vi "Stack_holderwise_total_bd_count_&_duration_ST1.vi"(0 "Refnum in":T1, 1 "BREAKDOWN_STK_HOLD_ID":i32=1, 2 "condition":string="Where BREAKDOWN_DATE between '%s'and '%s' and BREAKDOWN_STK_HOLD_ID ='%d'  ", 5 "Form Date":timestamp, 7 "Array":string[](array[string]), 9 "To Date":timestamp, 11 "error in (no error)":errorcluster, 12 "STATION_ID_CID_TRIGGER":i32, 13 "table":string[](array[string])=["STATION_1_LOG_HISTORY", "STATION_2_LOG_HISTORY", "STATION_3_LOG_HISTORY", "STATION_4_LOG_HISTORY", "STATION_5_LOG_HISTORY", "STATION_6_LOG_HISTORY"]) -> (4 "Refnum out":T1, 6 "Count out":string[](array[string]), 10 "appended array":dbl[](array[numeric]), 15 "error out":errorcluster)   [LabVIEW 2017]
uses:
  <vilib>/addons/database/Connection.llb/Conn ObjectReference.ctl
  <vilib>/addons/database/NI_Database_API.lvlib
panel:
  out "Table":string[][](array[string])
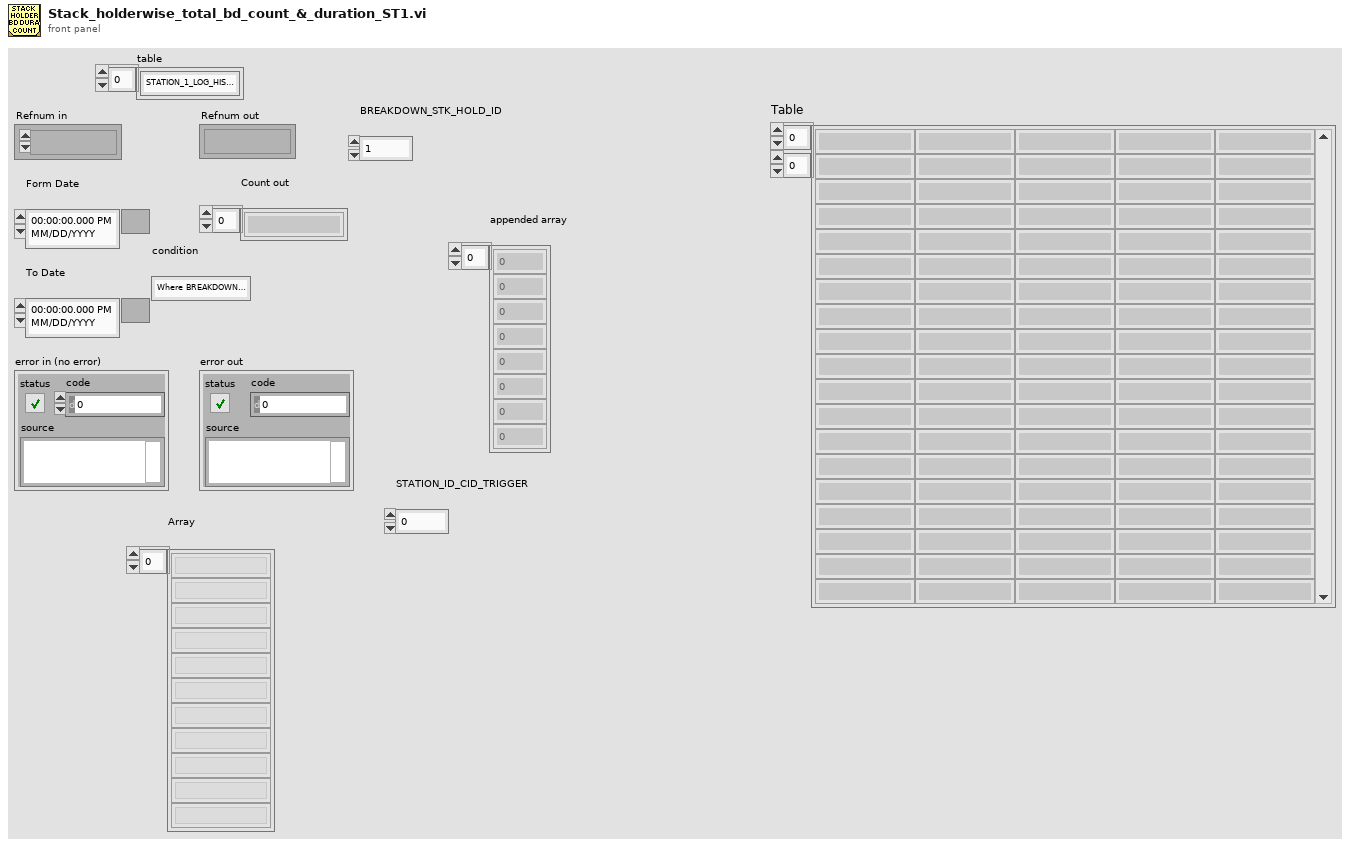
[diagram p1: front panel]
types:
  T1 = typedef "NI_Database_API.lvlib/Conn ObjectReference.ctl" = refnum<k1>
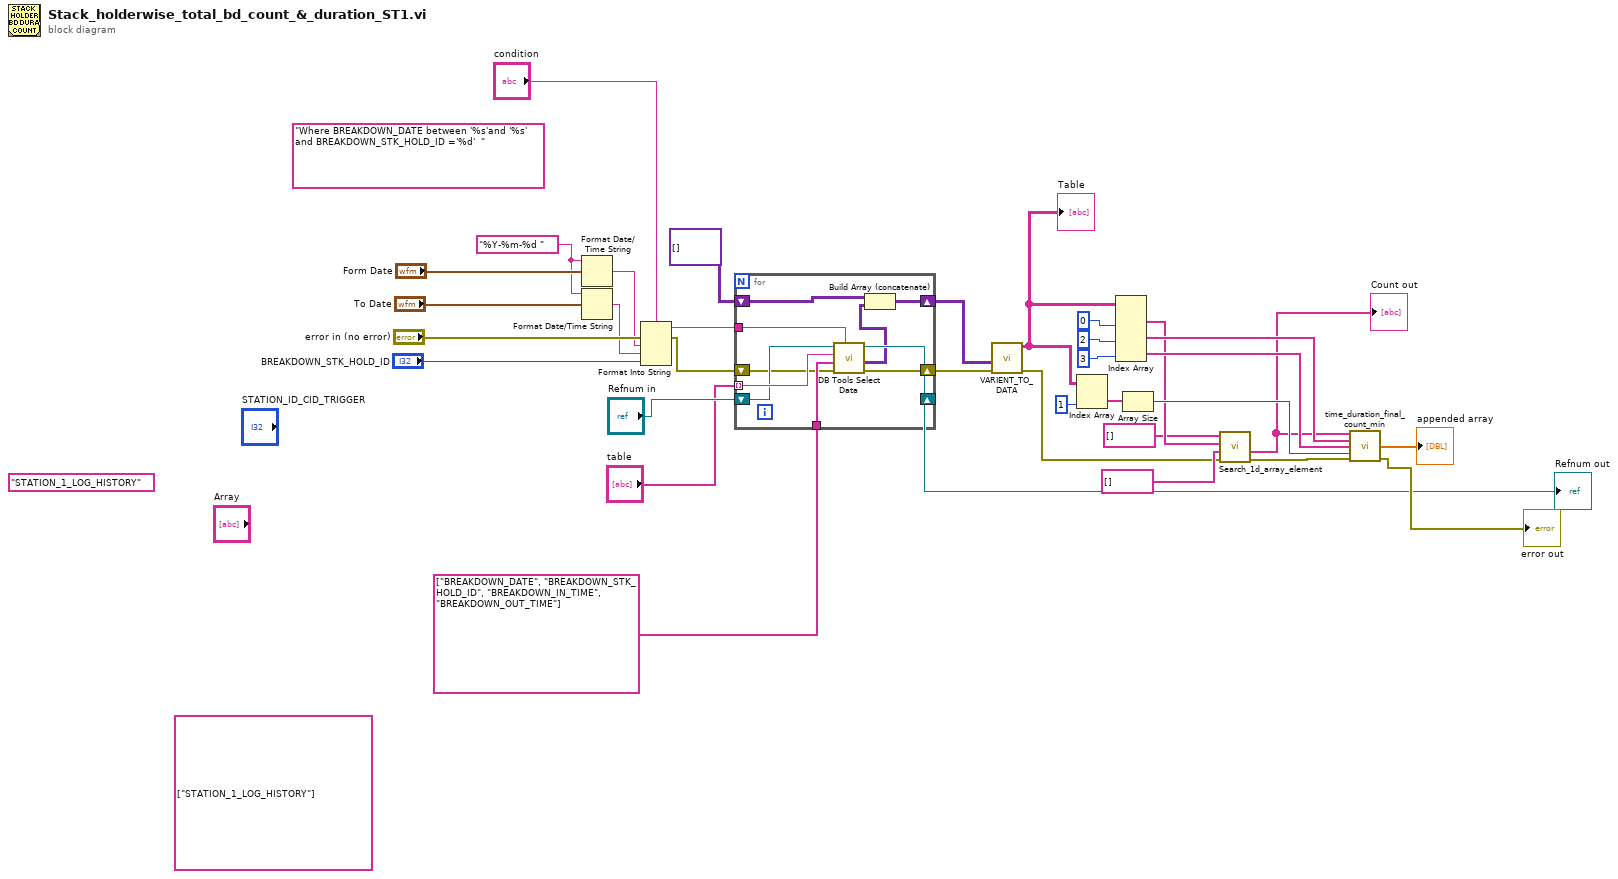
[diagram p0: block diagram]
diagram:
  (unwired) string[] ["STATION_1_LOG_HISTORY"]
  (unwired) "Where BREAKDOWN_DATE between '%s'and '%s' and BREAKDOWN_STK_HOLD_ID ='%d'  "
  (unwired) "STATION_1_LOG_HISTORY" ("table")
  w10 = "%Y-%m-%d " ("time format string (%c)")
  n1 = Format Date/Time String(time format string (%c)=w10, seconds (now)="Form Date") -> (date/time string=w13:string)  [unwired: 1 in]
  n2 = Format Date/Time String(time format string (%c)=w10, seconds (now)="To Date") -> (date/time string=w14:string)  [unwired: 1 in]
  n3 = Format Into String(format string="condition", error in="error in (no error)", w13, w14, "BREAKDOWN_STK_HOLD_ID") -> (resulting string=w6:string, error out=w7:errorcluster)  [unwired: 1 in]
  n4 = for {
    tunnel: "table" -> [w44] mode=indexing
    tunnel: string[] ["BREAKDOWN_DATE", "BREAKDOWN_STK_HOLD_ID", "BREAKDOWN_IN_TIME", "BREAKDOWN_OUT_TIME"] -> [w43]
    tunnel: w6 -> [w38]
    shift-right: [w42] -> w17
    shift-left: "Refnum in" -> [w41]
    shift-right: [w40] -> w8
    shift-left: w7 -> [w39]
    shift-right: [w35] -> w9
    shift-left: variant[][] [] ("data") -> [w37]
    n5 = call <vilib>:"DB Tools Select Data.vi"("condition"=w38, "error in (no error)"=w39, "columns"=w43, "table"=w44, "connection reference"=w41) -> ("error out"=w40:errorcluster, "data"=w36:variant[][], "connection reference out"=w42:T1)  [unwired: 1 in]
    n6 = Build Array (concatenate)(w37, w36) -> (w35:variant[][])
  }
  "Refnum out" <- w17
  n7 = call "VARIENT_TO_DATA.vi"("data"=w9, "error in (no error)"=w8) -> ("Table"=w31:string[][], "error out"=w32:errorcluster)  [unwired: 7 in]
  "Table" <- w31
  n8 = Index Array(array=w31, index (col)=1 ("disabled index (col)")) -> (element=w24:string[])  [unwired: 1 in]
  n9 = Index Array(array=w31, index (col) #1=0 ("disabled index (col)"), index (col) #2=2 ("disabled index (col)"), index (col) #3=3 ("disabled index (col)")) -> (element #1=w26:string[], element #2=w28:string[], element #3=w29:string[])  [unwired: 3 in]
  n10 = Array Size(array=w24) -> (size(s)=w30:i32)
  n11 = call "Search_1d_array_element.vi"("error in (no error)"=w32, "Count in"=string[] [] ("Count"), "BD Date"=w26, "Elements Found in"=string[] [] ("Elements Found")) -> ("error out"=w27:errorcluster, "Count out"=w5:string[])  [unwired: 3 in, 1 out]
  "Count out" <- w5
  n12 = call "time_duration_final_count_min.vi"("BD Count"=w5, "Intime"=w28, "OutTime"=w29, "bd array size"=w30, "error in (no error)"=w27) -> ("appended array"=→"appended array":dbl[], "error out"=→"error out":errorcluster)  [unwired: 7 in, 2 out]
